vi "ImageUpdateImage-1D.vi"(8 "error in (no error)":errorcluster, 10 "Data":dbl[][](array[numeric]), 11 "Image in":refnum<class "Image.lvclass">) -> (0 "error out":errorcluster, 2 "Image full":bool, 3 "Image out":refnum<class "Image.lvclass">)   [LabVIEW 2012, in "Image.lvclass"]
uses:
  classes/Image.lvclass
  classes/Image.lvclass/Image.ctl
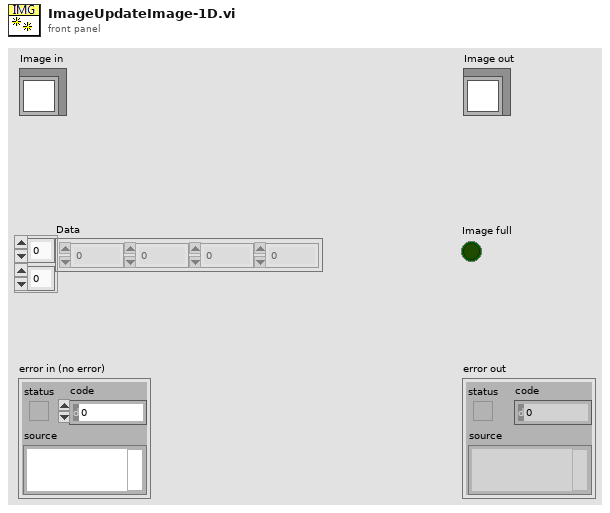
[diagram p1: front panel]
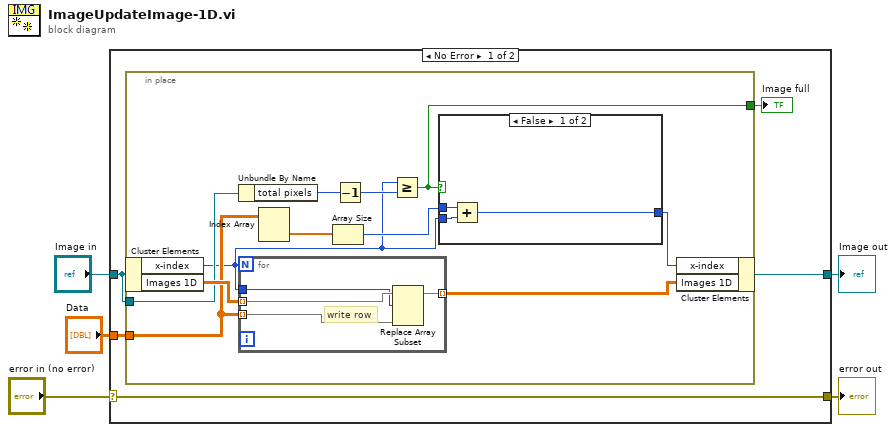
[diagram p0: block diagram]
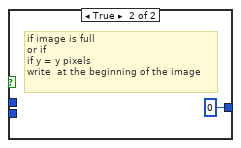
[diagram p2: hidden frame]
diagram:
  n1 = case shown="No Error" "error in (no error)" {
    selector: "error in (no error)" -> [w10 w31]
    tunnel: [w10 w31] -> w4
    tunnel: [w9 w30] -> w2
    tunnel: "Image in" -> [w6 w30]
    tunnel: "Data" -> [w8 _]
    frame No Error {
      n2 = in-place {
        in-place-border: w8 -> [w16]
        in-place-border: [w18] -> w7
        in-place-border: w6 -> [w13]
        n3 = in-place-cluster #1(w6) -> ("x-index"=w12:i32, "Images 1D"=w20:dbl[][][])
        n4 = Unbundle By Name(w13) -> ("total pixels"=w11:i32)
        n5 = for {
          tunnel: w20 -> [w25] mode=indexing
          tunnel: w16 -> [w24] mode=indexing
          tunnel: [w23] -> w19 mode=indexing
          tunnel: w12 -> [w22]
          # "write row"
          n6 = Replace Array Subset(array=w25, new element=w24, index (row)=w22) -> (w23:dbl[][])  [unwired: 1 in]
        }
        n7 = Index Array(array=w16) -> (element=w17:dbl[])  [unwired: 2 in]
        n8 = Array Size(array=w17) -> (size(s)=w15:i32)
        n9 = Decrement(x=w11) -> (x-1=w21:i32)
        n10 = Greater Or Equal?(x=w12, y=w21) -> (x >= y?=w18:bool)
        n11 = case shown="False" w18 {
          tunnel: w15 -> [w28 _]
          tunnel: w12 -> [w27 _]
          tunnel: [w26 0 ("t")] -> w14
          frame False {
            n12 = Add(x=w28, y=w27) -> (x+y=w26:i32)
          }
          frame True {
            # "if image is full\nor if\nif y = y pixels\nwrite  at the beginning of the image"
          }
        }
        n13 = in-place-cluster #1("x-index"=w14, "Images 1D"=w19) -> (w9:refnum<class "Image.lvclass">)
      }
      "Image full" <- w7
    }
    frame Error {
    }
  }
  "error out" <- w4
  "Image out" <- w2
